vi "GFITS_ReadAppendedHdrFiles.vi"(8 "error in":errorcluster, 10 "Path":path) -> (0 "error out":errorcluster, 1 "keywords found":i32, 2 "Array":string[][](array[string]))   [LabVIEW 2016]
panel:
  out "file names":string[](array[string])
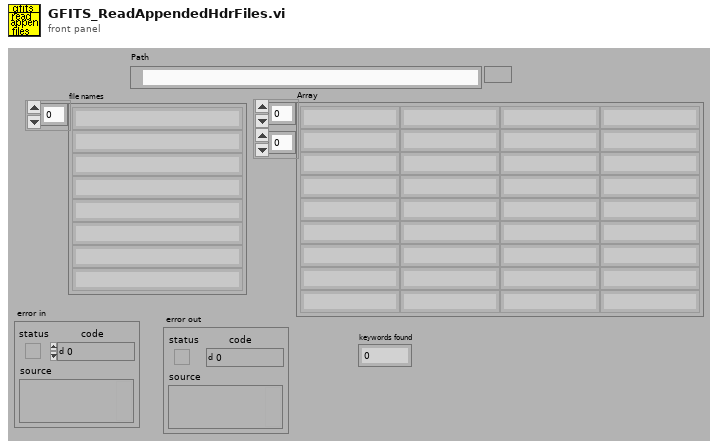
[diagram p1: front panel]
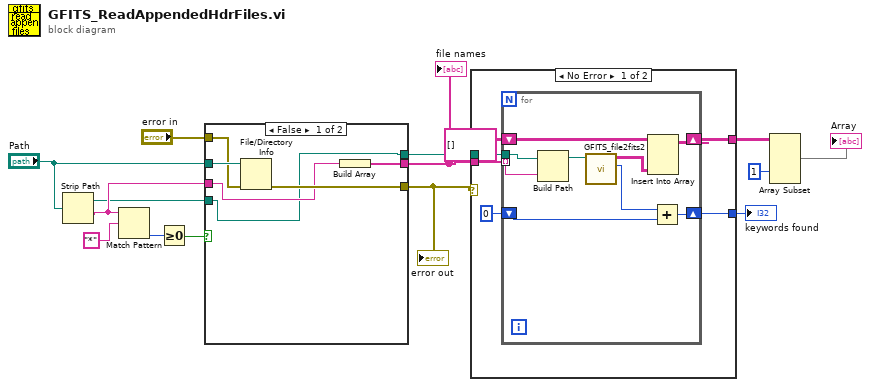
[diagram p0: block diagram]
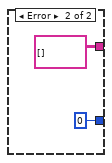
[diagram p2: hidden frame]
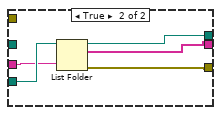
[diagram p3: hidden frame]
diagram:
  n1 = Strip Path(path="Path") -> (stripped path=w9:path, name=w11:string)
  n2 = Match Pattern(string=w11, regular expression="*") -> (offset past match=w13:i32)  [unwired: 4 out]
  n3 = Greater Or Equal To 0?(x=w13) -> (x >= 0?=w10:bool)
  n4 = case shown="False" w10 {
    tunnel: "Path" -> [w20 _]
    tunnel: w11 -> [w16 w24]
    tunnel: w9 -> [w15 w25]
    tunnel: [w19 w22] -> w7
    tunnel: [w18 w23] -> w6
    tunnel: "error in" -> [w17 _]
    tunnel: [w15 w21] -> w5
    frame False {
      n5 = File/Directory Info(path=w20, error in=w17) -> (error out=w19:errorcluster)  [unwired: 6 out]
      n6 = Build Array(w16) -> (w18:string[])
    }
    frame True {
      n7 = List Folder(path=w25, pattern=w24) -> (path out=w21:path, filenames=w23:string[], error out=w22:errorcluster)  [unwired: 1 in, 2 out]
    }
  }
  "file names" <- w6
  "error out" <- w7
  n8 = case shown="No Error" w7 {
    tunnel: w6 -> [w31 _]
    tunnel: [w30 string[][] []] -> w3
    tunnel: w5 -> [w28 _]
    tunnel: [w26 0] -> w4
    frame No Error {
      n9 = for {
        tunnel: w31 -> [w36] mode=indexing
        shift-right: [w39] -> w30
        shift-left: string[][] [] -> [w38]
        tunnel: w28 -> [w37]
        shift-right: [w33] -> w26
        shift-left: 0 -> [w32]
        n10 = Build Path(base path=w37, name or relative path=w36) -> (appended path=w35:path)
        n11 = call "GFITS_file2fits2.vi"("file"=w35) -> ("number of after keywords"=w34:i32, "after Keywords"=w40:string[][])  [unwired: 1 in, 8 out]
        n12 = Insert Into Array(array=w38, new element=w40) -> (w39:string[][])  [unwired: 2 in]
        n13 = Add(x=w34, y=w32) -> (x+y=w33:i32)
      }
    }
    frame Error {
    }
  }
  "keywords found" <- w4
  n14 = Array Subset(array=w3, index (col)=1 ("index")) -> (→"Array":string[][])  [unwired: 3 in]
